vi "Event Get Time.vi"(8 "error in (no error)":errorcluster, 11 "Event DVR in":refnum<data-value>) -> (0 "error out":errorcluster, 2 "Time out":refnum<data-value>, 3 "Event DVR out":refnum<data-value>)   [LabVIEW 2010, in "MDSplus.lvlib"]
doc: "Return last event reception time."
uses:
  <vilib>/MDSplus/Library/MDSplus.lvlib
  <vilib>/MDSplus/Classes/Event_Class/Event.lvclass
  <vilib>/MDSplus/Classes/Data_Class/Scalar_Class/Uint64_Class/Uint64.lvclass
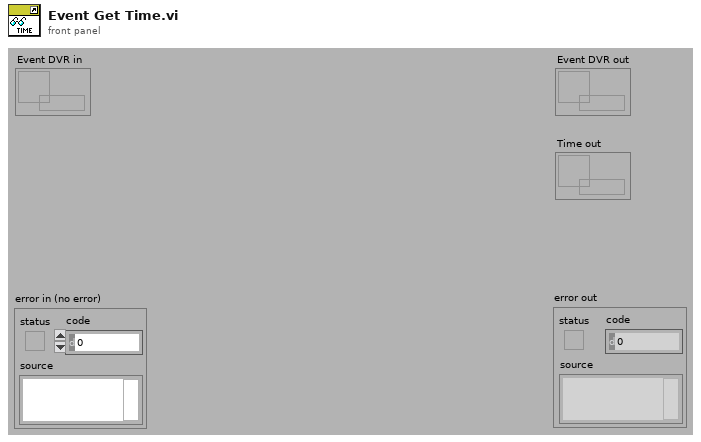
[diagram p1: front panel]
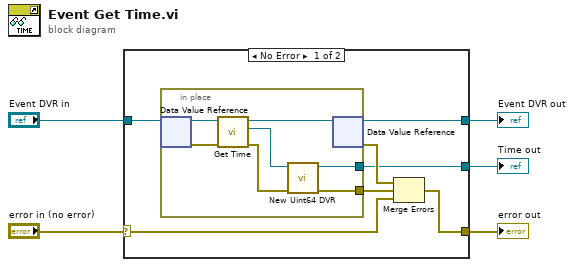
[diagram p0: block diagram]
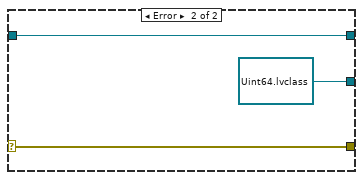
[diagram p2: hidden frame]
diagram:
  n1 = case shown="No Error" "error in (no error)" {
    selector: "error in (no error)" -> [w11 w22]
    tunnel: "Event DVR in" -> [w12 w21]
    tunnel: [w8 w22] -> w5
    tunnel: [w9 w21] -> w2
    tunnel: [w6 refnum<data-value> refnum ("Data DVR")] -> w1
    frame No Error {
      n2 = in-place {
        in-place-border: [w15] -> w6
        in-place-border: [w14] -> w7
        n3 = in-place-dvr #1(w12) -> (w19:refnum<class "Event.lvclass">, w18:errorcluster)
        n4 = call-dynamic "Get Time.vi"("error in (no error)"=w18, "Event in"=w19) -> ("error out"=w13:errorcluster, "Time out"=w16:refnum<class "Uint64.lvclass">, "Event out"=w17:refnum<class "Event.lvclass">)  [unwired: 7 in]
        n5 = call <vilib>:"New Uint64 DVR.vi"("error in (no error)"=w13, "Uint64 in"=w16) -> ("error out"=w14:errorcluster, "Uint64 DVR out"=w15:refnum<data-value>)  [unwired: 8 in]
        n6 = in-place-dvr #1(w17) -> (w9:refnum<data-value>, w10:errorcluster)
      }
      n7 = Merge Errors(w10, w7, w11) -> (w8:errorcluster)
    }
    frame Error {
    }
  }
  "error out" <- w5
  "Event DVR out" <- w2
  "Time out" <- w1
